vi "MFCCfinal.vi"() -> ()   [LabVIEW 2012]
uses:
  <vilib>/silver_ctls/ArrayMatrixCluster/Real Matrix NI_Silver.ctl
  <vilib>/Analysis/3filter.llb/FIR Filter (DBL).vi
  <vilib>/Analysis/baseanly.llb/Mean (DBL).vi
  <vilib>/Utility/file.llb/Read From Spreadsheet File (DBL).vi
  <vilib>/Analysis/2dsp.llb/Real FFT.vi
  <vilib>/Analysis/2dsp.llb/1D DCT.vi
  <vilib>/Utility/file.llb/Write To Spreadsheet File (DBL).vi
  <vilib>/Analysis/4window.llb/Hamming Window (DBL).vi
  <vilib>/Analysis/NI_AALBase.lvlib
  <vilib>/Analysis/NI_AALPro.lvlib
  <vilib>/Analysis/NI_AAL_SigProc.lvlib
panel:
  out "Rozpoznano":bool
  out "Min. wartość":dbl
  out "Min. indeks":i32
  out "Wynik":dbl[](array[numeric])
  out "Dane rozpoznawane":T1
  out "Dane zapisane":T1
  in  "Pomiar":bool=TRUE
  in  "Liczenie":bool
  out "Mowa wejściowa":waveform(dbl)[](graph)
  out "Częstotliwości środka":dbl[](array[numeric])
  out "Wypowiedź":dbl[](graph)
  out "Ind. końcowy":dbl
  out "Ind. początkowy":dbl
  out "\"Wygładzona\" energia":dbl[](graph)
  out "Długość":dbl
  out "Suma":dbl
  out "Wymiar":i32
  out "Diagram energii":dbl[](graph)
  out "Energia progowa":dbl
  out "Liczba wierszy":i32
  out "Liczba kolumn":i32
  out "Tablica ramek":dbl[](graph)
  out "Przekroczenie progu":bool
  out "Ramki":dbl[][](array[numeric])
  out "Energia sygnału":dbl
  in  "Stop":bool
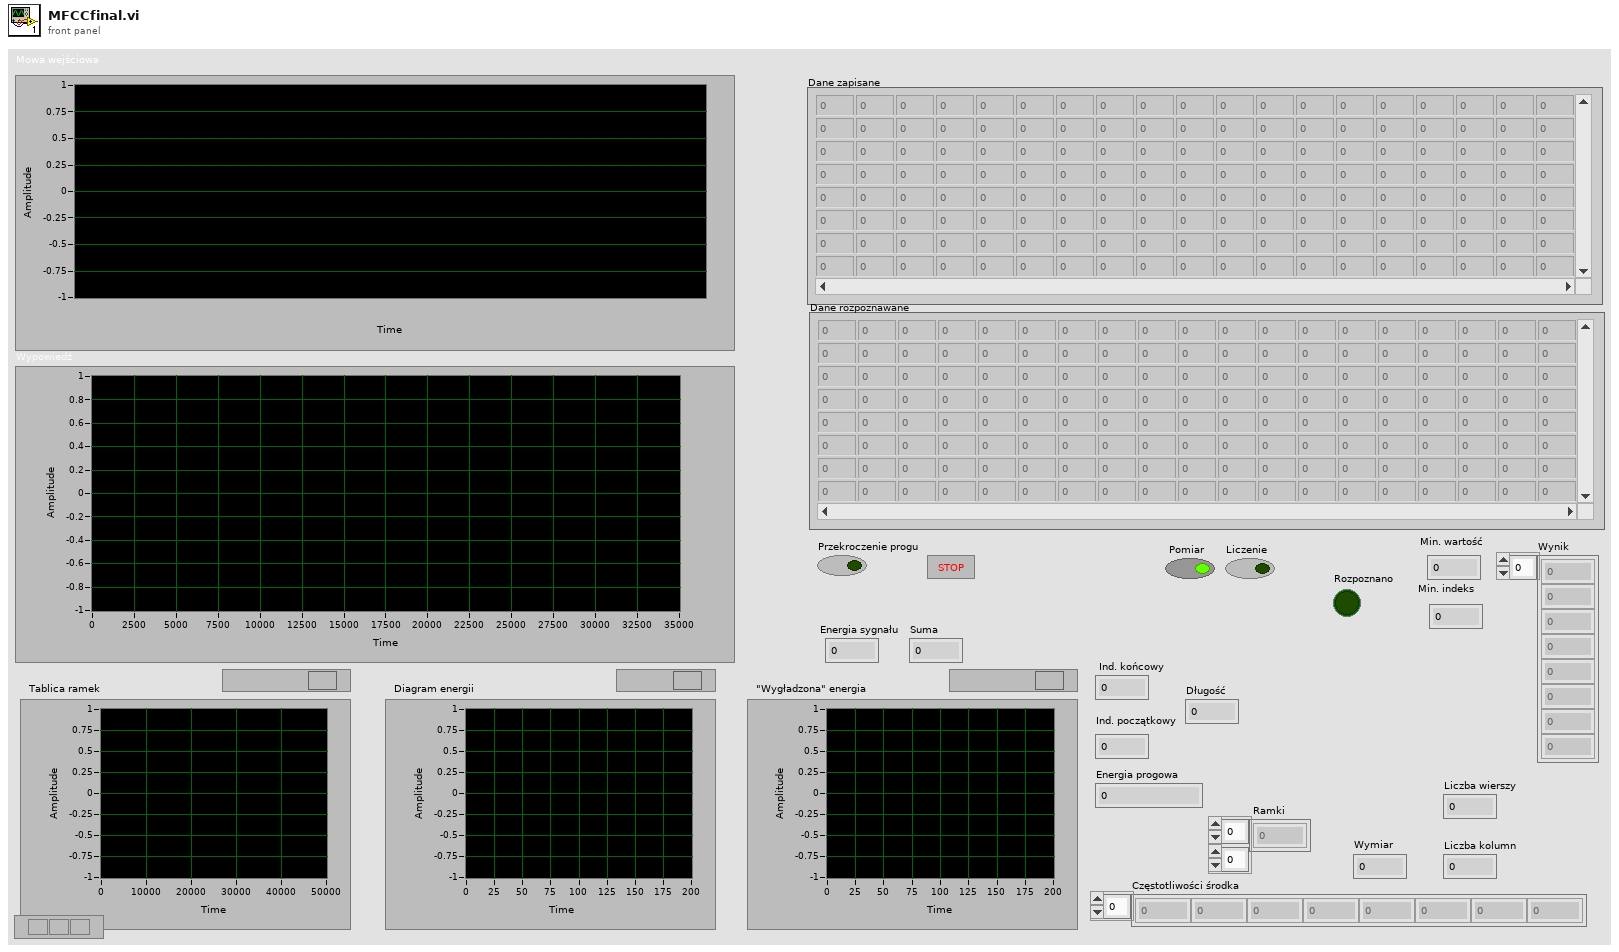
[diagram p1: front panel]
types:
  T1 = typedef "Real Matrix NI_Silver.ctl" = dbl[][]
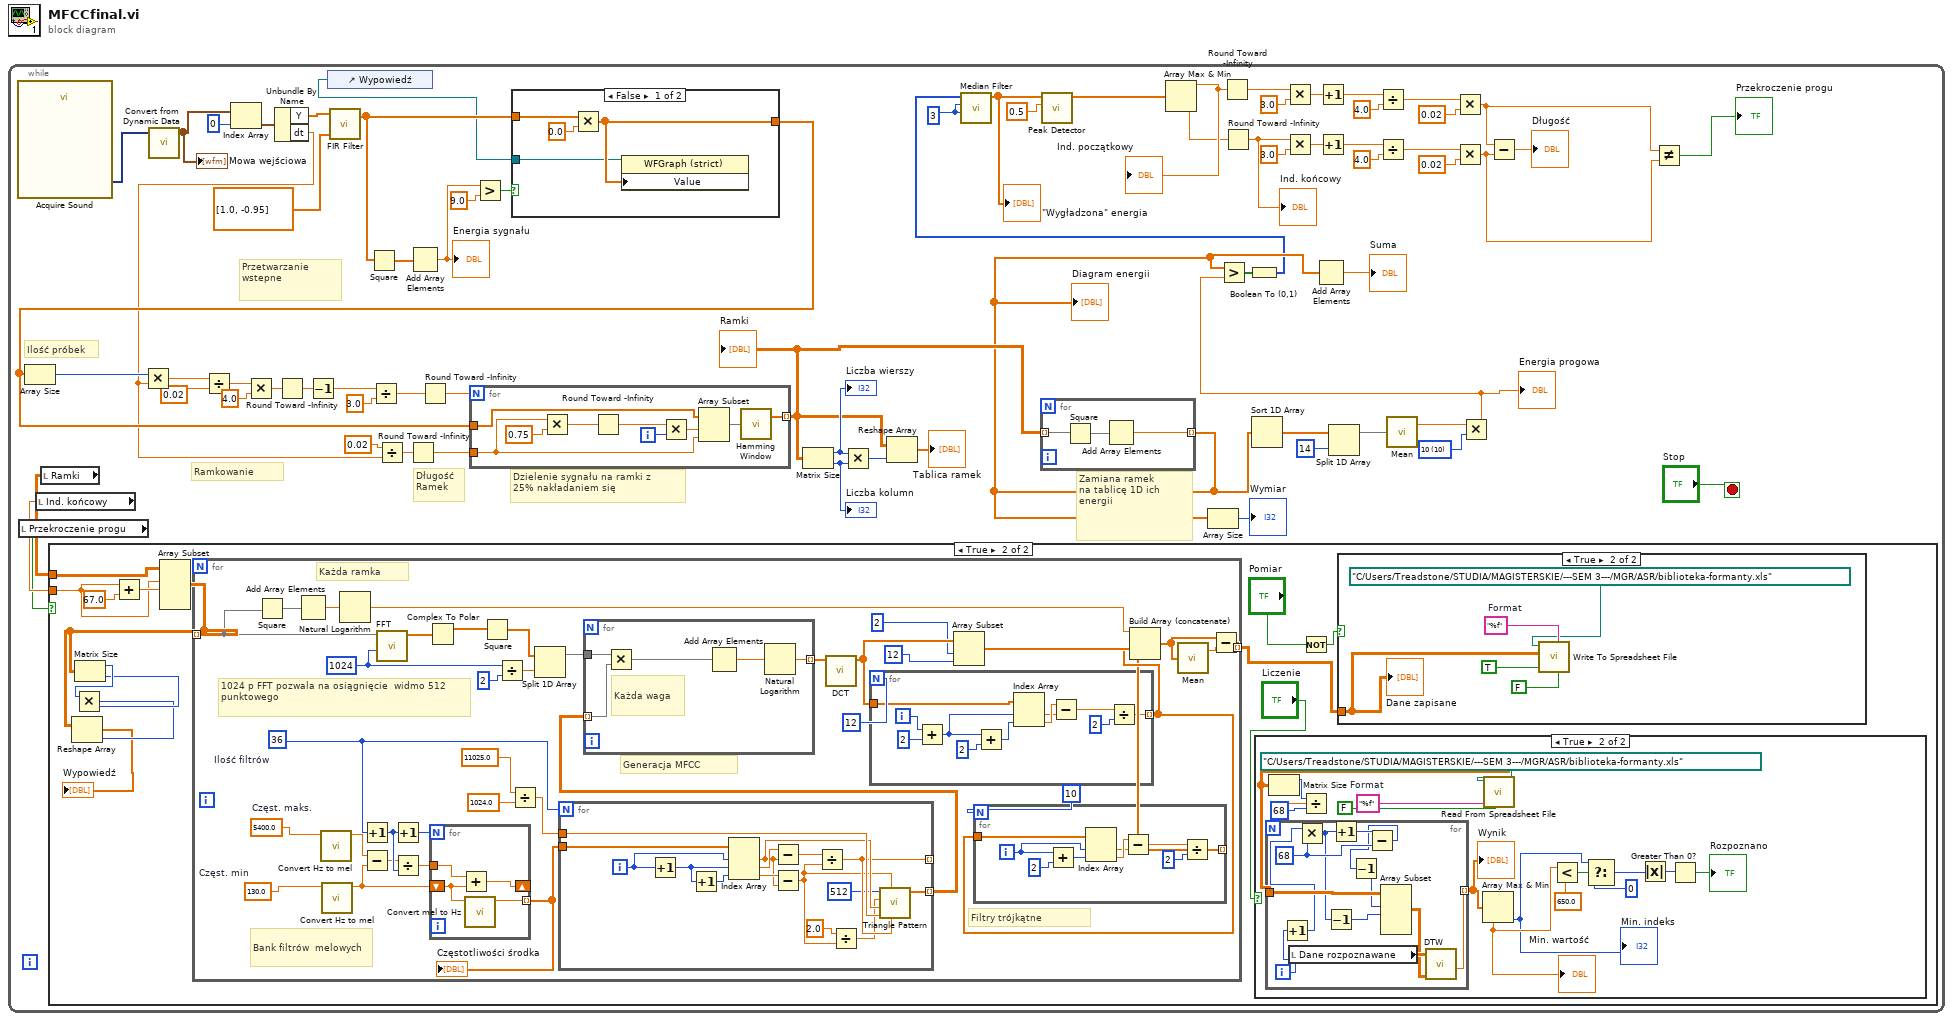
[diagram p0: block diagram]
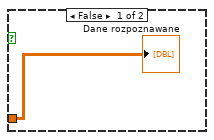
[diagram p3: hidden frame]
diagram:
  n1 = while {
    stop <- "Stop" stop-if-true
    w16 = 3 ("right rank")
    w40 = u16 10 items=["5"=5, "6"=6, "7"=7, "9"=9, "10"=10]
    # "Ramkowanie"
    # "Przetwarzanie \nwstepne"
    # "Zamiana ramek  \nna tablicę 1D ich \nenergii"
    # "Dzielenie sygnału na ramki z \n25% nakładaniem się"
    # "Długość\nRamek"
    # "Ilość próbek"
    n2 = call "Acquire Sound"() -> ("Data"=w72:dynamicdata)  [unwired: 18 in, 1 out]
    n3 = local read "Przekroczenie progu"() -> (w2:bool)
    n4 = local read "Ind. końcowy"() -> (w4:dbl)
    n5 = local read "Ramki"() -> (w3:dbl[][])
    n6 = case shown="True" w2 {
      tunnel: w4 -> [_ w79]
      tunnel: w3 -> [_ w80]
      frame False {
      }
      frame True {
        n7 = Add(x=w79, y=67.0 ("x")) -> (x+y=w84:dbl)
        n8 = Array Subset(array=w80, index (row)=w79, length (row)=w84) -> (w77:dbl[][])  [unwired: 2 in]
        n9 = Matrix Size(0:w77) -> (1:w83:i32, 2:w82:i32)
        n10 = Multiply(x=w83, y=w82) -> (x*y=w81:i32)
        n11 = Reshape Array(w77, w81) -> (→"Wypowiedź":dbl[])
        n12 = for {
          tunnel: w77 -> [w148] mode=indexing
          tunnel: [w123] -> w76 mode=indexing
          w152 = 1024 ("FFT size")
          w127 = 36  # Ilość filtrów
          w125 = 5400.0  # Częst. maks.
          w126 = 130.0  # Częst. min
          # "Filtry trójkątne"
          # "Bank filtrów  melowych"
          # "Każda ramka"
          # "Generacja MFCC"
          # "1024 p FFT pozwala na osiągnięcie  widmo 512  punktowego"
          n13 = Square(x=w148) -> (x^2=w147:dbl[])
          n14 = Add Array Elements(numeric array=w147) -> (sum=w146:dbl)
          n15 = call "Convert Hz to mel.vi"("Hz"=w125) -> ("mel"=w129:dbl)  [unwired: 10 in]
          n16 = call "Convert Hz to mel.vi"("Hz"=w126) -> ("mel"=w132:dbl)  [unwired: 10 in]
          n17 = Natural Logarithm(1:w146) -> (0:w142:dbl)
          n18 = Increment(x=w127) -> (x+1=w133:i32)
          n19 = Subtract(x=w129, y=w132) -> (x-y=w130:dbl)
          n20 = call-poly <vilib>:"FFT.vi"("FFT size"=w152, "X"=w148) -> ("FFT {X}"=w154:cdb[])  [unwired: 8 in, 1 out]
          n21 = Increment(x=w133) -> (x+1=w128:i32)
          n22 = Divide(x=w130, y=w133) -> (x/y=w131:dbl)
          n23 = Complex To Polar(r * e^(i*theta)=w154) -> (r=w153:dbl[])  [unwired: 1 out]
          n24 = for {
            N: w128 -> [_]
            tunnel: w131 -> [w173]
            tunnel: [w175] -> w137 mode=indexing
            shift-right: [w172] -> _
            shift-left: w132 -> [w174]
            n25 = Add(x=w173, y=w174) -> (x+y=w172:dbl)
            n26 = call "Convert mel to Hz.vi"("mel"=w174) -> ("Hz"=w175:dbl)  [unwired: 10 in]
          }
          "Częstotliwości środka" <- w137
          n27 = Square(x=w153) -> (x^2=w149:dbl[])
          n28 = Divide(x=w152, y=2 ("FFT size")) -> (x/y=w150:dbl)
          n29 = Divide(x=11025.0, y=1024.0) -> (x/y=w136:dbl)
          n30 = Split 1D Array(array=w149, index=w150) -> (first subarray=w156:dbl[])  [unwired: 1 out]
          n31 = for {
            N: w127 -> [_]
            tunnel: [w168] -> w124 mode=indexing
            tunnel: w137 -> [w167]
            tunnel: w136 -> [w166]
            tunnel: [w161] -> _ mode=indexing
            i -> [w171]
            n32 = Increment(x=w171) -> (x+1=w170:i32)
            n33 = Increment(x=w170) -> (x+1=w169:i32)
            n34 = Index Array(array=w167, index #1=w171, index #2=w170, index #3=w169) -> (element #1=w163:dbl, element #2=w164:dbl, element #3=w165:dbl)
            n35 = Subtract(x=w164, y=w163) -> (x-y=w162:dbl)
            n36 = Subtract(x=w165, y=w163) -> (x-y=w160:dbl)
            n37 = Divide(x=w162, y=w160) -> (x/y=w161:dbl)
            n38 = Divide(x=2.0, y=w160) -> (x/y=w158:dbl)
            n39 = call <vilib>:"Triangle Pattern.vi"("asymmetry"=w161, "width (s)"=w160, "delta t (s)"=w166, "delay (s)"=w163, "amplitude"=w158, "samples"=512) -> ("Triangle Pattern"=w168:dbl[])  [unwired: 4 in, 1 out]
          }
          n40 = for {
            tunnel: w124 -> [w199] mode=indexing
            tunnel: [w197] -> w155 mode=indexing
            tunnel: w156 -> [w196]
            # "Każda waga"
            n41 = Multiply(x=w196, y=w199) -> (x*y=w200:dbl[])
            n42 = Add Array Elements(numeric array=w200) -> (sum=w198:dbl)
            n43 = Natural Logarithm(1:w198) -> (0:w197:dbl)
          }
          n44 = call-poly <vilib>:"DCT.vi"("X"=w155) -> ("DCT {X}"=w144:dbl[])  [unwired: 9 in, 1 out]
          n45 = for {
            N: 12 -> [_]
            tunnel: w144 -> [w195]
            tunnel: [w188] -> w121 mode=indexing
            i -> [w193]
            n46 = Add(x=w193, y=2) -> (x+y=w185:i32)
            n47 = Add(x=w185, y=2) -> (x+y=w186:i32)
            n48 = Index Array(array=w195, index #1=w185, index #2=w186) -> (element #1=w191:dbl, element #2=w192:dbl)
            n49 = Subtract(x=w192, y=w191) -> (x-y=w190:dbl)
            n50 = Divide(x=w190, y=2) -> (x/y=w188:dbl)
          }
          n51 = Array Subset(array=w144, index=2, length=12 ("index")) -> (w141:dbl[])
          n52 = for {
            N: 10 -> [_]
            tunnel: w121 -> [w184]
            tunnel: [w178] -> w120 mode=indexing
            i -> [w177]
            n53 = Add(x=w177, y=2) -> (x+y=w176:i32)
            n54 = Index Array(array=w184, index #1=w177, index #2=w176) -> (element #1=w181:dbl, element #2=w182:dbl)
            n55 = Subtract(x=w182, y=w181) -> (x-y=w180:dbl)
            n56 = Divide(x=w180, y=2) -> (x/y=w178:dbl)
          }
          n57 = Build Array (concatenate)(w142, w141, w121, w120) -> (w139:dbl[])
          n58 = call-poly <vilib>:"Mean.vi"("X"=w139) -> ("mean"=w140:dbl)  [unwired: 1 out]
          n59 = Subtract(x=w139, y=w140) -> (x-y=w123:dbl[])
        }
        n60 = case shown="True" "Liczenie" {
          frame False {
          }
          frame True {
            w106 = "%f"  # Format
            n61 = call-poly <vilib>:"Read From Spreadsheet File.vi"("transpose (no:F)"=FALSE, "format (%.3f)"=w106, "file path (dialog if empty)"=path "C:/Users/Treadstone/STUDIA/MAGISTERSKIE/---SEM 3---/MGR/ASR/biblioteka-formanty.xls") -> ("all rows"=w102:dbl[][])  [unwired: 4 in, 4 out]
            n62 = Matrix Size(0:w102) -> (1:w104:i32)  [unwired: 1 out]
            n63 = Divide(x=w104, y=68) -> (x/y=w101:dbl)
            n64 = for {
              N: w101 -> [_]
              tunnel: w102 -> [w116]
              tunnel: [w113] -> w100 mode=indexing
              i -> [w111]
              w118 = 68
              n65 = Increment(x=w111) -> (x+1=w110:i32)
              n66 = local read "Dane rozpoznawane"() -> (w115:T1)
              n67 = Multiply(x=w110, y=w118) -> (x*y=w112:i32)
              n68 = Decrement(x=w112) -> (x-1=w108:i32)
              n69 = Increment(x=w112) -> (x+1=w119:i32)
              n70 = Subtract(x=w119, y=w118) -> (x-y=w117:i32)
              n71 = Decrement(x=w117) -> (x-1=w109:i32)
              n72 = Array Subset(array=w116, index (row)=w109, length (row)=w108) -> (w114:dbl[][])  [unwired: 2 in]
              n73 = call "DTW.vi"("Reference Sequence"=w114, "Test Sequence"=w115) -> ("Cost"=w113:dbl)  [unwired: 9 in]
            }
            "Wynik" <- w100
            n74 = Array Max & Min(array=w100) -> (min value=w98:dbl, min index (indices)=w97:i32)  [unwired: 2 out]
            "Min. indeks" <- w97
            "Min. wartość" <- w98
            n75 = Less?(x=w98, y=650.0) -> (x < y?=w99:bool)
            n76 = Select(t=w97, s=w99, f=0) -> (s? t:f=w95:i32)
            n77 = Absolute Value(x=w95) -> (abs(x)=w94:i32)
            n78 = Greater Than 0?(x=w94) -> (x > 0?=→"Rozpoznano":bool)
          }
        }
        n79 = Not(x="Pomiar") -> (.not. x?=w73:bool)
        n80 = case shown="True" w73 {
          tunnel: w76 -> [w86 w88]
          frame False {
            "Dane rozpoznawane" <- w86
          }
          frame True {
            w91 = "%f"  # Format
            n81 = call-poly <vilib>:"Write To Spreadsheet File.vi"("transpose? (no:F)"=FALSE, "format (%.3f)"=w91, "append to file? (new file:F)"=TRUE, "2D data"=w88, "file path (dialog if empty)"=path "C:/Users/Treadstone/STUDIA/MAGISTERSKIE/---SEM 3---/MGR/ASR/biblioteka-formanty.xls") -> ()  [unwired: 3 in, 1 out]
            "Dane zapisane" <- w88
          }
        }
      }
    }
    n82 = call "Convert from Dynamic Data"("Dynamic Data Type"=w72) -> ("Array of Waveform"=w1:waveform(dbl)[])  [unwired: 3 in]
    "Mowa wejściowa" <- w1
    n83 = Index Array(array=w1, index=0) -> (element=w62:waveform(dbl))
    n84 = Unbundle By Name(w62) -> ("Y"=w61:dbl[], "dt"=w41:dbl)
    n85 = control-ref of="Wypowiedź"() -> (w5:refnum<vi>)
    n86 = call-poly <vilib>:"FIR Filter.vi"("FIR Coefficients"=dbl[] [1.0, -0.95], "X"=w61) -> ("Filtered X"=w70:dbl[])  [unwired: 2 in, 1 out]
    n87 = Square(x=w70) -> (x^2=w66:dbl[])
    n88 = Divide(x=0.02, y=w41) -> (x/y=w47:dbl)
    n89 = Round Toward -Infinity(1:w47) -> (0:w48:dbl)
    n90 = Add Array Elements(numeric array=w66) -> (sum=w68:dbl)
    "Energia sygnału" <- w68
    n91 = Greater?(x=w68, y=9.0) -> (0:w69:bool)
    n92 = case shown="False" w69 {
      tunnel: w70 -> [w215 w217]
      tunnel: [w214 w217] -> w42
      tunnel: w5 -> [w213 _]
      frame False {
        n93 = Multiply(x=w215, y=0.0) -> (x*y=w214:dbl[])
        n94 = property class="WFGraph (strict)"(reference=w213, "Value"=w214) -> ()  [unwired: 1 in, 2 out]
      }
      frame True {
      }
    }
    n95 = Array Size(array=w42) -> (size(s)=w60:i32)
    n96 = Multiply(x=w60, y=w41) -> (x*y=w58:dbl)
    n97 = Divide(x=w58, y=0.02) -> (x/y=w54:dbl)
    n98 = Multiply(x=w54, y=4.0) -> (x*y=w53:dbl)
    n99 = Round Toward -Infinity(1:w53) -> (0:w56:dbl)
    n100 = Decrement(x=w56) -> (x-1=w51:dbl)
    n101 = Divide(x=w51, y=3.0) -> (x/y=w50:dbl)
    n102 = Round Toward -Infinity(1:w50) -> (0:w49:dbl)
    n103 = for {
      N: w49 -> [_]
      tunnel: w42 -> [w212]
      tunnel: w48 -> [w209]
      tunnel: [w204] -> w32 mode=indexing
      i -> [w211]
      n104 = Multiply(x=w209, y=0.75 ("x")) -> (x*y=w207:dbl)
      n105 = Round Toward -Infinity(1:w207) -> (0:w206:dbl)
      n106 = Multiply(x=w206, y=w211) -> (x*y=w208:dbl)
      n107 = Array Subset(array=w212, index=w208, length=w209) -> (w205:dbl[])
      n108 = call-poly <vilib>:"Hamming Window.vi"("X"=w205) -> ("Windowed X"=w204:dbl[])  [unwired: 1 out]
    }
    "Ramki" <- w32
    n109 = Matrix Size(0:w32) -> (1:w46:i32, 2:w45:i32)
    "Liczba kolumn" <- w45
    "Liczba wierszy" <- w46
    n110 = Multiply(x=w46, y=w45) -> (x*y=w44:i32)
    n111 = Reshape Array(w32, w44) -> (→"Tablica ramek":dbl[])
    n112 = for {
      tunnel: w32 -> [w203] mode=indexing
      tunnel: [w201] -> w9 mode=indexing
      n113 = Square(x=w203) -> (x^2=w202:dbl[])
      n114 = Add Array Elements(numeric array=w202) -> (sum=w201:dbl)
    }
    "Diagram energii" <- w9
    n115 = Array Size(array=w9) -> (size(s)=→"Wymiar":i32)
    n116 = Sort 1D Array(array=w9) -> (sorted array=w36:dbl[])
    n117 = Add Array Elements(numeric array=w9) -> (sum=→"Suma":dbl)
    n118 = Split 1D Array(array=w36, index=14) -> (first subarray=w34:dbl[])  [unwired: 1 out]
    n119 = call-poly <vilib>:"Mean.vi"("X"=w34) -> ("mean"=w33:dbl)  [unwired: 1 out]
    n120 = Multiply(x=w33, y=w40) -> (x*y=w39:dbl)
    "Energia progowa" <- w39
    n121 = Greater?(x=w9, y=w39) -> (0:w38:bool[])
    n122 = Boolean To (0,1)(Boolean=w38) -> (0, 1=w6:i16[])
    n123 = call <vilib>:"Median Filter.vi"("right rank"=w16, "left rank"=w16, "X"=w6) -> ("Filtered X"=w13:dbl[])  [unwired: 7 in, 1 out]
    "\"Wygładzona\" energia" <- w13
    n124 = call <vilib>:"Peak Detector.vi"("threshold"=0.5, "X"=w13) -> ("Locations"=w15:dbl[])  [unwired: 5 in, 4 out]
    n125 = Array Max & Min(array=w15) -> (max value=w17:dbl, min value=w12:dbl)  [unwired: 2 out]
    "Ind. początkowy" <- w17
    n126 = Round Toward -Infinity(1:w17) -> (0:w30:dbl)
    n127 = Round Toward -Infinity(1:w12) -> (0:w11:dbl)
    "Ind. końcowy" <- w11
    n128 = Multiply(x=w30, y=3.0) -> (x*y=w19:dbl)
    n129 = Multiply(x=w11, y=3.0) -> (x*y=w28:dbl)
    n130 = Increment(x=w19) -> (x+1=w20:dbl)
    n131 = Increment(x=w28) -> (x+1=w27:dbl)
    n132 = Divide(x=w20, y=4.0) -> (x/y=w22:dbl)
    n133 = Divide(x=w27, y=4.0) -> (x/y=w25:dbl)
    n134 = Multiply(x=w22, y=0.02) -> (x*y=w8:dbl)
    n135 = Multiply(x=w25, y=0.02) -> (x*y=w7:dbl)
    n136 = Subtract(x=w8, y=w7) -> (x-y=→"Długość":dbl)
    n137 = Not Equal?(x=w8, y=w7) -> (x != y?=→"Przekroczenie progu":bool)
  }
